vi "UpdateRobotModeVariables.vi"(11 "Frequency":dbl) -> ()   [LabVIEW 2014]
uses:
  <vilib>/Rock Robotics/WPI/DriverStation/WPI_DriverStationRobotMode2.ctl
  Variables/Default global.vi
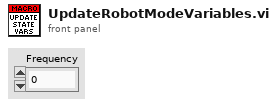
[diagram p1: front panel]
types:
  T1 = typedef "WPI_DriverStationRobotMode2.ctl" = enum16{"Autonomous Disabled", "Autonomous Enabled", "Teleop Disabled", "Teleop Enabled", "Disconnected", "Finish", "Test Disabled", "Test Enabled", "Emergency Stopped"}
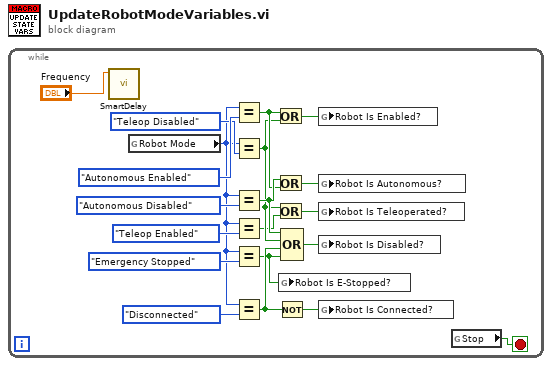
[diagram p0: block diagram]
diagram:
  n1 = while {
    stop <- w20 stop-if-true
    n2 = call "SmartDelay.vi"("Frequency"="Frequency") -> ()  [unwired: 11 in]
    n3 = global read "Default global.vi" "Robot Mode"() -> (w12:T1)
    n4 = Equal?(x=w12, y=WPI_DriverStationRobotMode2."Autonomous Enabled") -> (x = y?=w6:bool)
    n5 = Equal?(x=w12, y=WPI_DriverStationRobotMode2."Teleop Disabled") -> (x = y?=w4:bool)
    n6 = Equal?(x=w12, y=WPI_DriverStationRobotMode2."Autonomous Disabled") -> (x = y?=w10:bool)
    n7 = Equal?(x=w12, y=WPI_DriverStationRobotMode2."Teleop Enabled") -> (x = y?=w3:bool)
    n8 = Equal?(x=w12, y=WPI_DriverStationRobotMode2."Emergency Stopped") -> (x = y?=w1:bool)
    n9 = Equal?(x=w12, y=WPI_DriverStationRobotMode2."Disconnected") -> (x = y?=w8:bool)
    n10 = Or(x=w6, y=w4) -> (x .or. y?=w5:bool)
    n11 = Or(x=w10, y=w6) -> (x .or. y?=w11:bool)
    n12 = Or(x=w4, y=w3) -> (x .or. y?=w2:bool)
    n13 = Not(x=w8) -> (.not. x?=w7:bool)
    n14 = global write "Default global.vi" "Robot Is E-Stopped?"(w1) -> ()
    n15 = Compound Arithmetic op=OR(w10, w4, w8, w1) -> (w9:bool)
    n16 = global write "Default global.vi" "Robot Is Enabled?"(w5) -> ()
    n17 = global write "Default global.vi" "Robot Is Autonomous?"(w11) -> ()
    n18 = global write "Default global.vi" "Robot Is Teleoperated?"(w2) -> ()
    n19 = global write "Default global.vi" "Robot Is Disabled?"(w9) -> ()
    n20 = global write "Default global.vi" "Robot Is Connected?"(w7) -> ()
    n21 = global read "Default global.vi" "Stop"() -> (w20:bool)
  }
